vi "Read TOML File.vi"   [LabVIEW 2019, in "BlueTOMLSerializer.lvlib"]
uses:
  BlueTOMLSerializer.lvlib
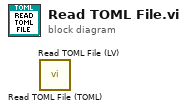
[diagram p0: block diagram]
diagram:
  n1 = call "Read TOML File (TOML).vi"() -> ()  [unwired: 10 in, 2 out]
  n2 = call "Read TOML File (LV).vi"() -> ()  [unwired: 10 in, 2 out]
